vi "test_ReservedName_CheckPluginNameIsValid_NameInvalid.vi"() -> (6 "pass":bool, 8 "result":string, 15 "error out":errorcluster)   [LabVIEW 2021]
uses:
  <vilib>/ErrorRing/Error Ring.xnode
  Generator/_Editor/MeasurementService Editor.lvlib
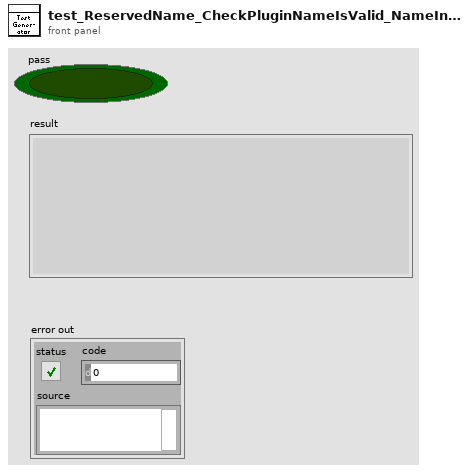
[diagram p1: front panel]
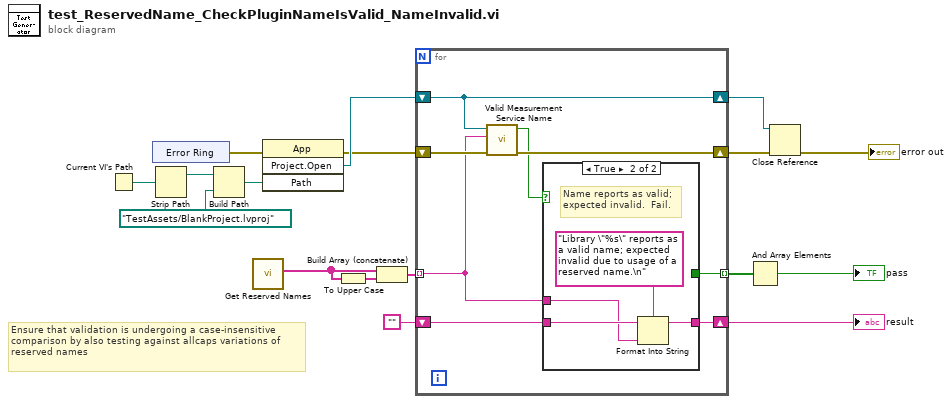
[diagram p0: block diagram]
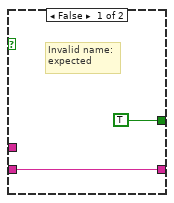
[diagram p2: hidden frame]
diagram:
  # "Ensure that validation is undergoing a case-insensitive comparison by also testing against allcaps variations of reserved names"
  n1 = Current VI's Path() -> (path=w17:path)
  n2 = xnode "Error Ring"() -> ("error out"=w14:errorcluster)
  n3 = Strip Path(path=w17) -> (stripped path=w16:path)  [unwired: 1 out]
  n4 = Build Path(base path=w16, name or relative path=path "TestAssets/BlankProject.lvproj" ("path")) -> (appended path=w13:path)
  n5 = call "Get Reserved Names.vi"() -> ("reserved names"=w1:string[])  [unwired: 11 in]
  n6 = invoke class="App" method="Project.Open"(error in=w14, "Path"=w13) -> (error out=w11:errorcluster, "Project:Open"=w12:refnum<vi>)  [unwired: 2 in, 2 out]
  n7 = To Upper Case(1:w1) -> (0:w2:string[])
  n8 = Build Array (concatenate)(w1, w2) -> (w3:string[])
  n9 = for {
    shift-right: [w24] -> w10
    shift-left: w11 -> [w25]
    tunnel: w3 -> [w18] mode=indexing
    shift-right: [w23] -> w8
    shift-left: w12 -> [w23]
    shift-right: [w20] -> w6
    shift-left: "" -> [w21]
    tunnel: [w19] -> w5 mode=indexing
    n10 = call "Valid Measurement Service Name.vi"("error in"=w25, "requested plugin name"=w18, "project ref"=w23) -> ("error out"=w24:errorcluster, "valid name?"=w22:bool)  [unwired: 7 in]
    n11 = case shown="True" w22 {
      tunnel: w21 -> [w27 w31]
      tunnel: [w27 w30] -> w20
      tunnel: [TRUE _] -> w19
      tunnel: w18 -> [_ w29]
      frame False {
        # "Invalid name:\nexpected"
      }
      frame True {
        # "Name reports as valid;\nexpected invalid.  Fail."
        n12 = Format Into String(format string="Library \"%s\" reports as a valid name; expected invalid due to usage of a reserved name.\n", initial string=w31, w29) -> (resulting string=w30:string)  [unwired: 1 in, 1 out]
      }
    }
  }
  "result" <- w6
  n13 = And Array Elements(Boolean array=w5) -> (logical AND=→"pass":bool)
  n14 = Close Reference(reference=w8, error in (no error)=w10) -> (error out=→"error out":errorcluster)
